vi "Control (1).vi"(0 "Cluster":T1, 1 "Current Temperature":dbl, 2 "error in":errorcluster) -> (3 "Heater on":bool, 4 "error out":errorcluster, 5 "Cooler On":bool, 6 "error out 2":errorcluster caption="error out")   [LabVIEW 2015]
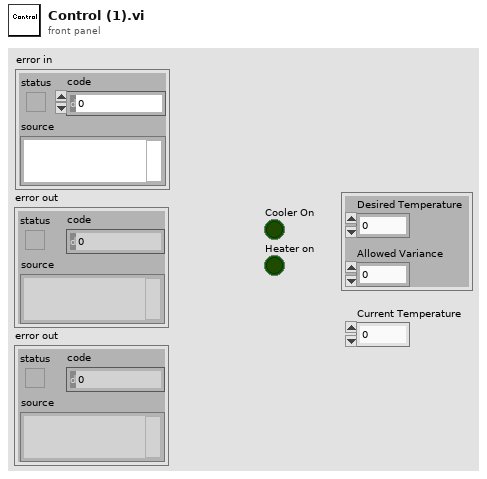
[diagram p1: front panel]
types:
  T1 = cluster{"Desired Temperature":dbl, "Allowed Variance":dbl}
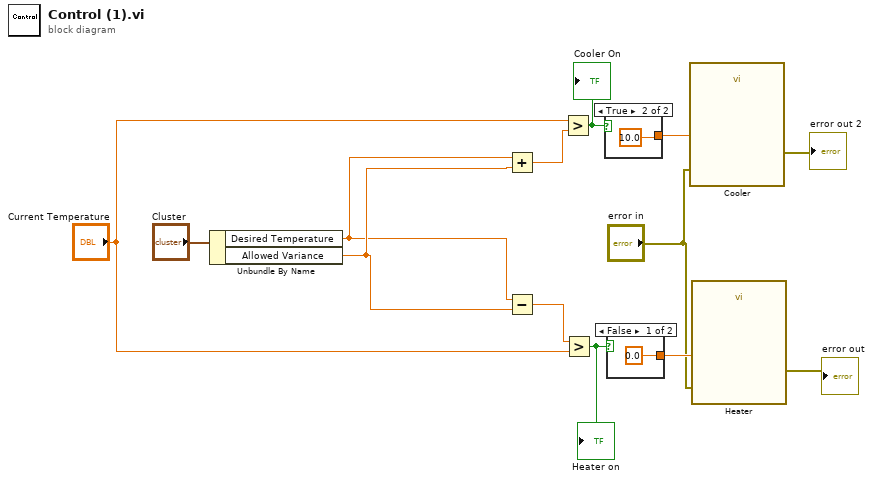
[diagram p0: block diagram]
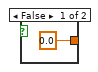
[diagram p2: hidden frame]
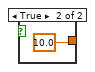
[diagram p3: hidden frame]
diagram:
  n1 = Unbundle By Name("Cluster") -> ("Desired Temperature"=w9:dbl, "Allowed Variance"=w10:dbl)
  n2 = Add(x=w9, y=w10) -> (x+y=w13:dbl)
  n3 = Subtract(x=w9, y=w10) -> (x-y=w12:dbl)
  n4 = Greater?(x="Current Temperature", y=w13) -> (0:w6:bool)
  "Cooler On" <- w6
  n5 = Greater?(x=w12, y="Current Temperature") -> (0:w8:bool)
  "Heater on" <- w8
  n6 = case shown="True" w6 {
    tunnel: [0.0 10.0 ("data")] -> w5
    frame False {
    }
    frame True {
    }
  }
  n7 = case shown="False" w8 {
    tunnel: [0.0 10.0 ("data")] -> w7
    frame False {
    }
    frame True {
    }
  }
  n8 = call "Cooler"("data"=w5, "error in"="error in") -> ("error out"=→"error out 2":errorcluster)  [unwired: 16 in, 1 out]
  n9 = call "Heater"("data"=w7, "error in"="error in") -> ("error out"=→"error out":errorcluster)  [unwired: 16 in, 1 out]
